vi "Get Device by Type Model.vi"(8 "error in (no error)":errorcluster, 9 "Model":string, 10 "Type":string, 11 "HAL Editor in":refnum<class "HAL Editor.lvclass">) -> (0 "error out":errorcluster, 2 "Device":refnum<class "Device.lvclass">, 3 "HAL Editor out":refnum<class "HAL Editor.lvclass">)   [LabVIEW 2012, in "HAL Config.lvlib" / "HAL Editor.lvclass"]
uses:
  HAL Editor.lvclass
  build/ppl/lv-hal.lvlibp/Device/Device.lvclass
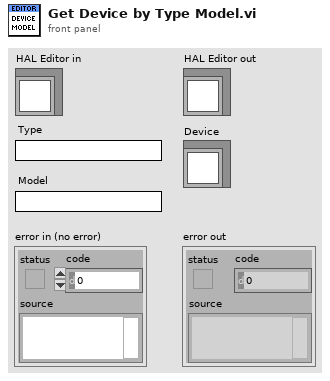
[diagram p1: front panel]
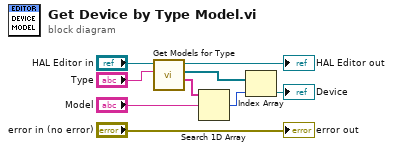
[diagram p0: block diagram]
diagram:
  n1 = call "Get Models for Type.vi"("Type"="Type", "HAL Editor in"="HAL Editor in") -> ("Models"=w6:string[], "Devices"=w4:refnum<class "Device.lvclass">[], "HAL Editor out"=→"HAL Editor out":refnum<class "HAL Editor.lvclass">)  [unwired: 6 in, 1 out]
  n2 = Search 1D Array(1D array=w6, element="Model") -> (index of element=w3:i32)  [unwired: 1 in]
  n3 = Index Array(array=w4, index=w3) -> (element=→"Device":refnum<class "Device.lvclass">)
  "error out" <- "error in (no error)"
